vi "update table.vi"(5 "Sort By...":T3 items=["RIO device", "resource", "input type", "datatype", "reserver"], 7 "selected values":bool[](array[boolean]), 8 "error in (no error)":errorcluster, 9 "Show":T1, 10 "MulticolumnListbox in":refnum<vi>, 11 "Item Ref in":T2 format="%.0x") -> (0 "error out":errorcluster, 3 "resource entries":T4[](array[typedef]) {"FPGA CD Ref" format="%.0x"; "reserver" format="%.0x"})   [LabVIEW 2016, in "RM.Server.lvlib"]
uses:
  RM.Server.lvlib
  viz_entry.ctl
  <vilib>/NI Veristand/Custom Device API/Custom Device Item Ref.ctl
  viz_type.ctl
  viz_show.ctl
  Shared/Global Tags.vi
  Shared/RM.Shared.lvlib
  <vilib>/NI Veristand/Custom Device API/Custom Device API.lvlib
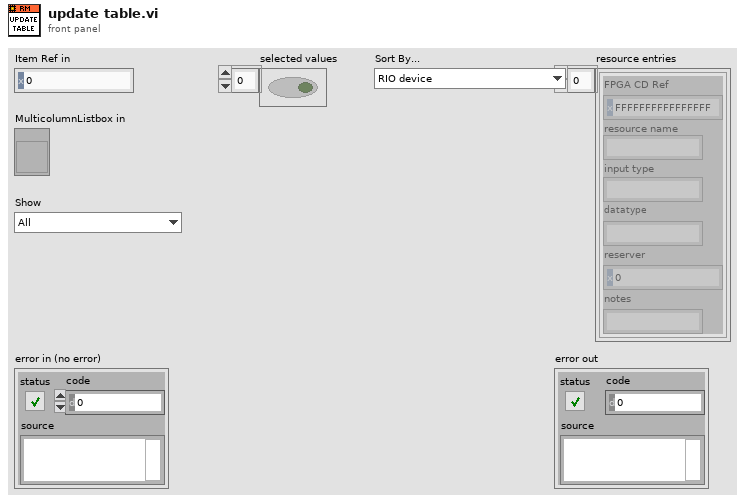
[diagram p1: front panel]
types:
  T1 = typedef "RM.Server.lvlib/viz_show.ctl" = enum16{"All", "Mapped", "Unmapped"}
  T2 = typedef "Custom Device API.lvlib/Custom Device Item Ref.ctl" = u64
  T3 = typedef "RM.Server.lvlib/viz_type.ctl" = u16
  T4 = typedef "RM.Server.lvlib/viz_entry.ctl" = cluster{"FPGA CD Ref":T2, "resource name":string, "input type":string, "datatype":string, "reserver":T2, "notes":string}
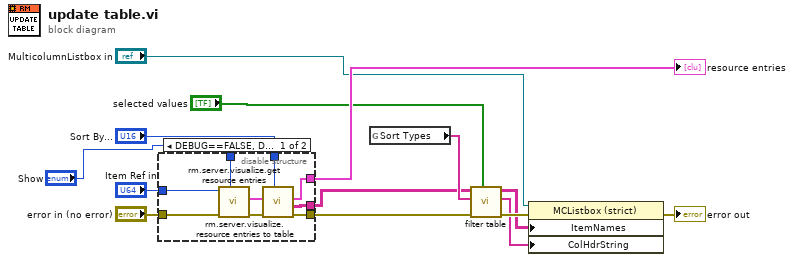
[diagram p0: block diagram]
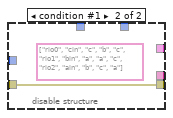
[diagram p2: hidden frame]
diagram:
  n1 = disable-structure shown="DEBUG==FALSE, Default" {
    disable-tunnel: "error in (no error)" -> [w23 w25]
    disable-tunnel: "Item Ref in" -> [w22 _]
    disable-tunnel: [w19 w25] -> w13
    disable-tunnel: [w17 _] -> w11
    disable-tunnel: "Show" -> [w18 _]
    disable-tunnel: [w16 _] -> w2
    disable-tunnel: "Sort By..." -> [w15 _]
    frame condition #0 (active) {
      n2 = call "rm.server.visualize.get resource entries.vi"("Show"=w18, "error in (no error)"=w23, "Item Ref in"=w22) -> ("error out"=w20:errorcluster, "resource entries"=w21:T4[])  [unwired: 6 in, 1 out]
      n3 = call "rm.server.visualize.resource entries to table.vi"("Sort Type"=w15, "error in (no error)"=w20, "resource entries"=w21) -> ("error out"=w19:errorcluster, "sorted resource table out"=w16:string[][], "sorted resource entries out"=w17:T4[])  [unwired: 6 in]
    }
    frame condition #1 {
      w24 = string[][] [["rio0", "cin", "c", "b", "c"], ["rio1", "bin", "a", "a", "c"], ["rio2", "ain", "b", "c", "a"]] ("resource table")
    }
  }
  "resource entries" <- w11
  n4 = global read "Global Tags.vi" "Sort Types"() -> (w12:string[])
  n5 = call "filter table.vi"("display column?"="selected values", "error in (no error)"=w13, "Sort Types"=w12, "resource table in"=w2) -> ("error out"=w14:errorcluster, "Headers"=w9:string[], "resource table out"=w10:string[][])  [unwired: 5 in]
  n6 = property on="Property Node" class="MCListbox (strict)"(reference="MulticolumnListbox in", error in=w14, "ItemNames"=w10, "ColHdrString"=w9) -> (error out=→"error out":errorcluster)  [unwired: 1 out]
